vi "Set Motors Position Setpoint.vi"(8 "error in (no error)":errorcluster, 10 "position (m)":dbl[](array[numeric])=[0.0, 0.0, 0.0, 0.0, 0.0], 11 "KUKA youBot gripper in":refnum<class "NI_Robotics_KUKA youBot Gripper.lvclass">) -> (0 "error out":errorcluster, 3 "KUKA youBot gripper out":refnum<class "NI_Robotics_KUKA youBot Gripper.lvclass">)   [LabVIEW 2017, in "NI_Robotics_KUKA youBot Host.lvlib" / "NI_Robotics_KUKA youBot Gripper.lvclass"]
doc: "Sets the position setpoint of the motors attached to the joints of a KUKA youBot gripper."
uses:
  <vilib>/robotics/KUKA youBot/Basic Device/Gripper/NI_Robotics_KUKA youBot Gripper.lvclass
  <vilib>/robotics/KUKA youBot/Basic Device/Gripper/NI_Robotics_KUKA youBot Gripper.lvclass/NI_Robotics_KUKA youBot Gripper.ctl
  <vilib>/robotics/KUKA youBot/Motor/Gripper Motor/NI_Robotics_KUKA youBot Gripper Motor.lvclass
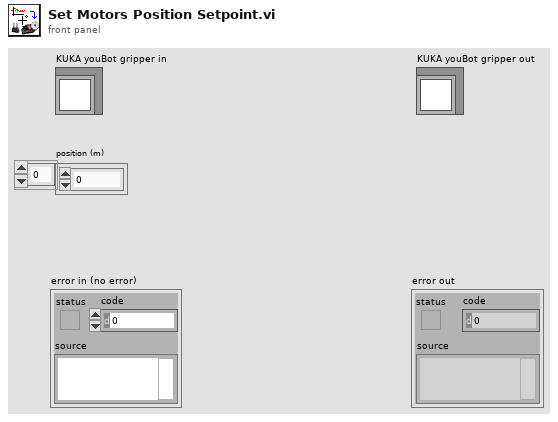
[diagram p1: front panel]
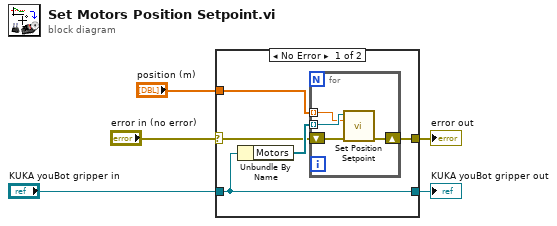
[diagram p0: block diagram]
diagram:
  n1 = case shown="No Error" "error in (no error)" {
    selector: "error in (no error)" -> [w7 w16]
    tunnel: [w6 w16] -> w4
    tunnel: [w10 w15] -> w2
    tunnel: "KUKA youBot gripper in" -> [w10 w15]
    tunnel: "position (m)" -> [w8 _]
    frame No Error {
      n2 = Unbundle By Name(w10) -> ("Motors"=w9:refnum<class "NI_Robotics_KUKA youBot Gripper Motor.lvclass">[])
      n3 = for {
        tunnel: w9 -> [w14] mode=indexing
        tunnel: w8 -> [w13] mode=indexing
        shift-right: [w11] -> w6
        shift-left: w7 -> [w12]
        n4 = call-dynamic "Set Position Setpoint.vi"("error in (no error)"=w12, "position (m)"=w13, "KUKA youBot gripper motor in"=w14) -> ("error out"=w11:errorcluster)  [unwired: 7 in, 1 out]
      }
    }
    frame Error {
    }
  }
  "error out" <- w4
  "KUKA youBot gripper out" <- w2
